vi "2 Element Array FXP(+-,14,1) to I16.vi"(0 "data in":fxp<+/-,14,1>[](array[numeric])=[0.0, 0.0]) -> (4 "data out":i16[](array[numeric]), 6 "overflow":bool)   [LabVIEW 2015]
doc: "Converts data type from one format to another. The acceptable data types are: +- FXP 18,1; +-, FXP 14,1; and I16.\n\n<B>Supported data types</B>\nFXP +-,18,1; FXP +-,14,1; I16\n\n<B>Supported channel size</B>\n4, 8\n\n<B>Supported samples per cycle</B>\n2\n\n<B>Input Parameters</B>\n\n<B>data in</B> specifies the data to convert to another data type.\n\n<B>Output Parameters</B>\n\n<B>data out</B> returns the converted data.\n\n<B>overflow</B> returns the overflow carried through the data path."
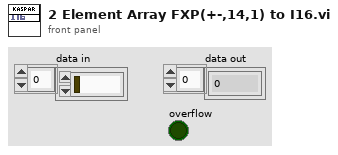
[diagram p1: front panel]
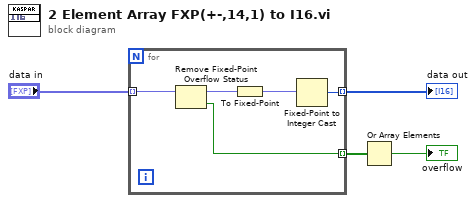
[diagram p0: block diagram]
diagram:
  n1 = for {
    tunnel: "data in" -> [w9] mode=indexing
    tunnel: [w6] -> w3 mode=indexing
    tunnel: [w5] -> w2 mode=indexing
    n2 = Remove Fixed-Point Overflow Status(3:w9) -> (0:w6:bool, 1:w8:fxp<+/-,14,1>)
    n3 = To Fixed-Point(number=w8) -> (fixed-point=w7:fxp<+/-,16,1>)  [unwired: 1 in]
    n4 = Fixed-Point to Integer Cast(1:w7) -> (0:w5:i16)
  }
  "data out" <- w2
  n5 = Or Array Elements(Boolean array=w3) -> (logical OR=→"overflow":bool)
